vi "AudioStreamer.Get Error Message.vi"() -> (0 "message":string)   [LabVIEW 2020]
uses:
  <vilib>/Utility/error.llb/DialogType.ctl
  Typedefs/AudioStreamer.Globals.vi
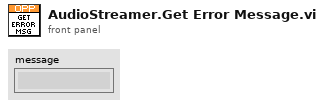
[diagram p1: front panel]
types:
  T1 = typedef "DialogType.ctl" = u16
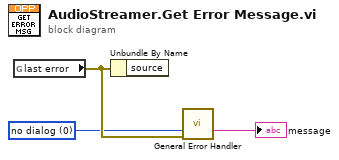
[diagram p0: block diagram]
diagram:
  w2 = T1 0 items=["no dialog", "OK message", "continue or stop message", "OK message + warnings", "continue/stop + warnings"] ("type of dialog (OK msg:1)")
  n1 = global read "AudioStreamer.Globals.vi" "last error"() -> (w3:errorcluster)
  n2 = Unbundle By Name(w3) -> ()  [unwired: 1 out]
  n3 = call <vilib>:"General Error Handler.vi"("type of dialog (OK msg:1)"=w2, "error in (no error)"=w3) -> ("message"=→"message":string)  [unwired: 9 in, 4 out]
